vi "Store Multicarrier Setup Information.vi"(8 "error in (no error)":errorcluster, 10 "Stored File Name":string, 11 "VISA resource name":refnum<visa-resource-name>) -> (0 "error out":errorcluster, 3 "VISA resource name out":refnum<visa-resource-name>)   [LabVIEW 2018, in "Agilent PSG MXG Series.lvlib"]
doc: "Stores the current multicarrier setup information to a file.\nThe stored file contains information that includes the digital modulation format, number of carriers, frequency spacing, and power settings for the multicarrier setup.\n\n<b>Note:</b>\nIt is applicable for N5172B/82B with <b>Option 431</b>, or N5162A, N5182A."
uses:
  Agilent PSG MXG Series.lvlib
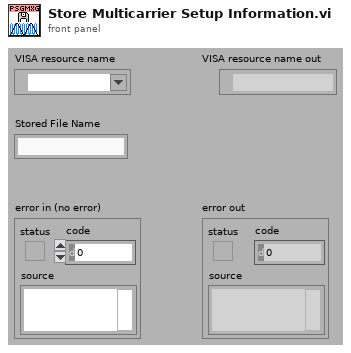
[diagram p1: front panel]
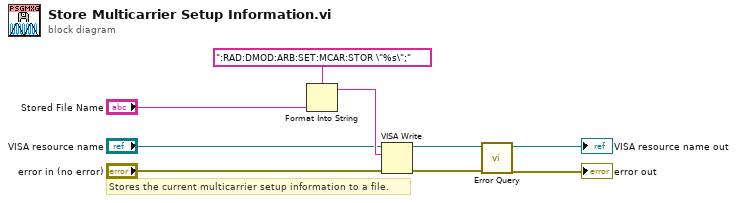
[diagram p0: block diagram]
diagram:
  # "Stores the current multicarrier setup information to a file."
  n1 = Format Into String(format string=":RAD:DMOD:ARB:SET:MCAR:STOR \"%s\";", "Stored File Name") -> (resulting string=w7:string)  [unwired: 2 in, 1 out]
  n2 = VISA Write(VISA resource name="VISA resource name", write buffer=w7, error in (no error)="error in (no error)") -> (VISA resource name out=w4:refnum<visa-resource-name>, error out=w3:errorcluster)  [unwired: 1 out]
  n3 = call "Error Query.vi"("error in (no error)"=w3, "VISA resource name"=w4) -> ("error out"=→"error out":errorcluster, "VISA resource name out"=→"VISA resource name out":refnum<visa-resource-name>)  [unwired: 6 in, 2 out]
